vi "Query Current Range.vi"(8 "error in (no error)":errorcluster, 11 "VISA resource name":refnum<visa-resource-name>) -> (0 "error out":errorcluster, 1 "Maximum value":u16, 2 "Minimum value":u16, 3 "VISA resource name out":refnum<visa-resource-name>)   [LabVIEW 2013, in "IT6900.lvlib"]
doc: "Provides the range of values for query current."
uses:
  IT6900.lvlib
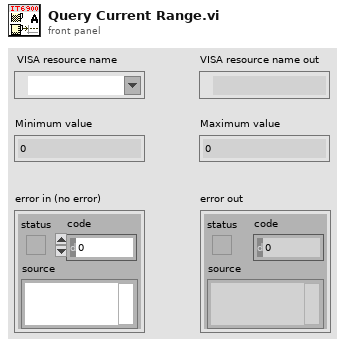
[diagram p1: front panel]
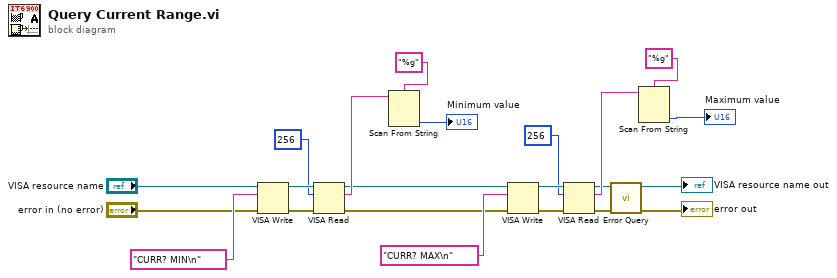
[diagram p0: block diagram]
diagram:
  n1 = VISA Write(VISA resource name="VISA resource name", write buffer="CURR? MIN\n", error in (no error)="error in (no error)") -> (VISA resource name out=w18:refnum<visa-resource-name>, error out=w19:errorcluster)  [unwired: 1 out]
  n2 = VISA Read(VISA resource name=w18, byte count=256, error in (no error)=w19) -> (VISA resource name out=w8:refnum<visa-resource-name>, read buffer=w16:string, error out=w7:errorcluster)  [unwired: 1 out]
  n3 = Scan From String(format string="%g", input string=w16) -> (output 1=→"Minimum value":u16)  [unwired: 3 in, 3 out]
  n4 = VISA Write(VISA resource name=w8, write buffer="CURR? MAX\n", error in (no error)=w7) -> (VISA resource name out=w11:refnum<visa-resource-name>, error out=w12:errorcluster)  [unwired: 1 out]
  n5 = VISA Read(VISA resource name=w11, byte count=256, error in (no error)=w12) -> (VISA resource name out=w3:refnum<visa-resource-name>, read buffer=w9:string, error out=w4:errorcluster)  [unwired: 1 out]
  n6 = call "Error Query.vi"("error in (no error)"=w4, "VISA resource name"=w3) -> ("error out"=→"error out":errorcluster, "VISA resource name out"=→"VISA resource name out":refnum<visa-resource-name>)  [unwired: 6 in, 2 out]
  n7 = Scan From String(format string="%g", input string=w9) -> (output 1=→"Maximum value":u16)  [unwired: 3 in, 3 out]
